vi "FTW-ExtendedActorTemplate.vi"(0 "FTW Actor Instance Configuration":string="{\n  \"Identity\": \"ActorName\",\n  \"InboxAddress\": \"inproc://*\",\n  \"LoggerAddress\": \"\",\n  \"DebugEnableInboxLogging\": false,\n  \"DebugEnableJobLogging\": false,\n  \"LauncherAddress\": \"\",\n  \"Connections\": {\n    \"ConnectionOne\": \"inproc://connection-one\",\n    \"ConnectionTwo\": \"tcp://localhost/connection-two\"\n  },\n  \"Publishers\": {\n    \"PublisherOne\": \"inproc://publisher-one\",\n    \"PublisherTwo\": \"tcp://localhost/publisher-two\"\n  },\n  \"Subscriptions\": {\n    \"SubscriptionOne\": \"inproc://subscription-one\",\n    \"SubscriptionTwo\": \"tcp://localhost/subscription-two\"\n  }\n}", 11 "ErrorIn":errorcluster) -> (15 "Error":errorcluster)   [LabVIEW 2013]
uses:
  source/actor/Instance-Extended/FTW-ActorExtended.lvclass
  source/actor/Message/Base/FTW-Message.lvclass
  source/actor/Instance/FTW-ActorInstance.lvclass/FTW-ActorInstance.ctl
  source/actor/JobSequencer/FTW-SEQ-Current.vi
  source/actor/Instance/FTW-ActorInstance.lvclass
  source/actor/Message/Request/FTW-Message-IncomingRequest.lvclass
panel:
  # "Inputs"
  # "Outputs"
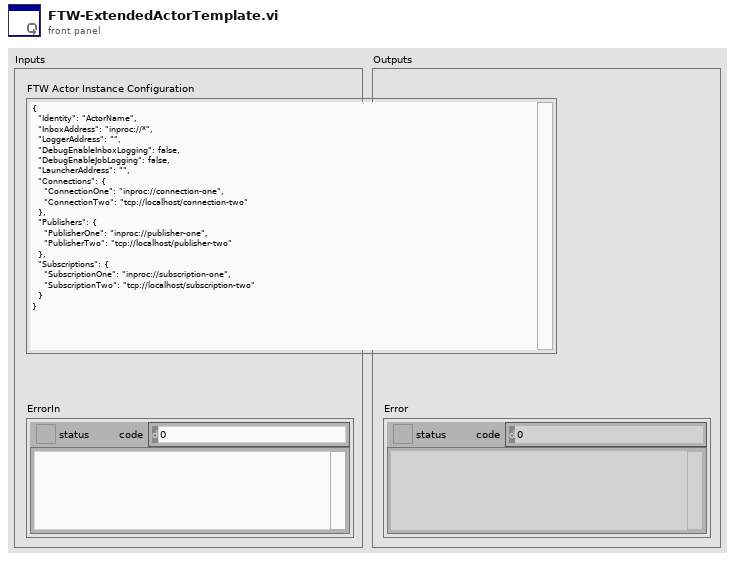
[diagram p1: front panel]
types:
  T1 = cluster{"Incoming Requests":refnum<event-registration>, "Local Messages":refnum<event-registration>, "Subscriber Registration":refnum<event-registration>}
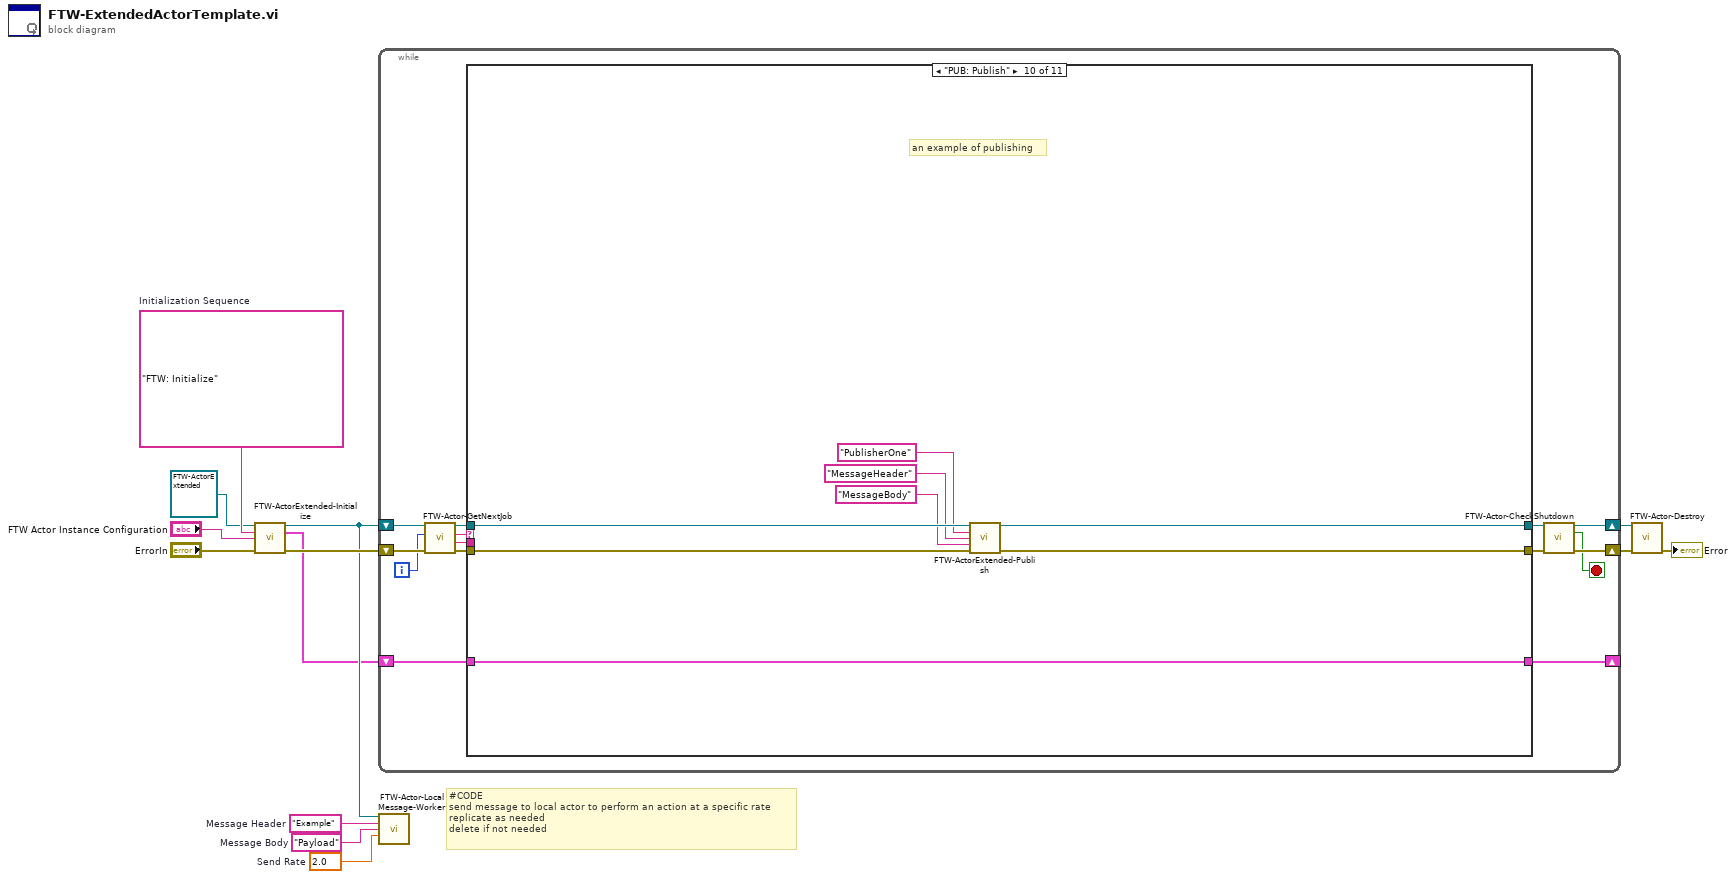
[diagram p0: block diagram]
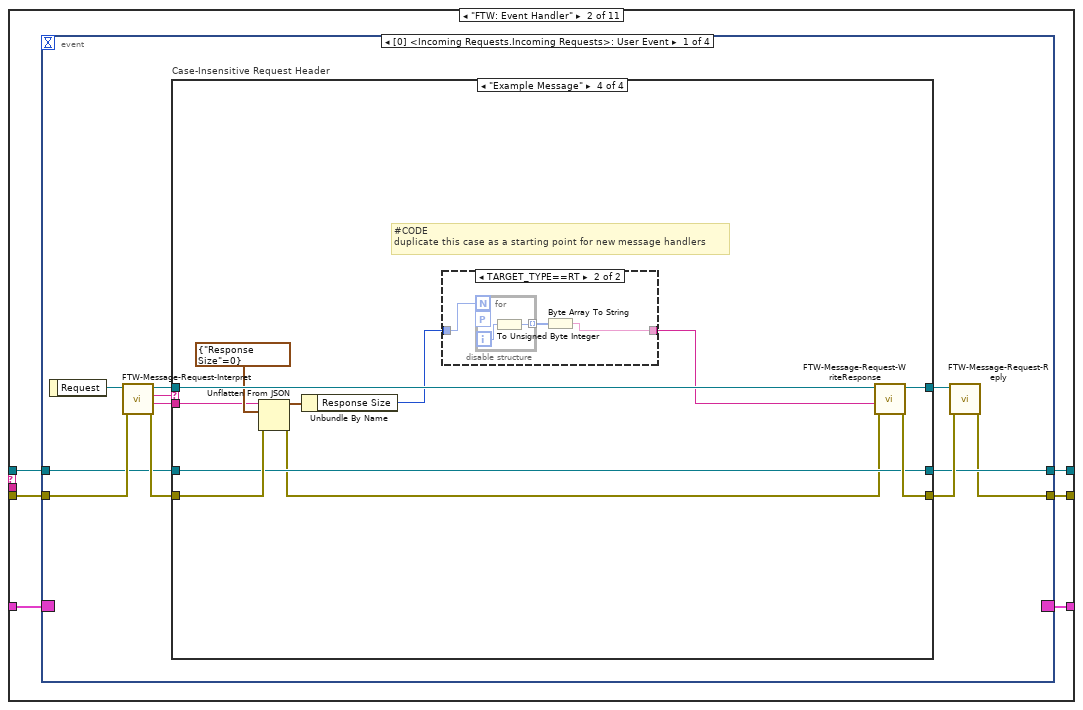
[diagram p3: hidden frame]
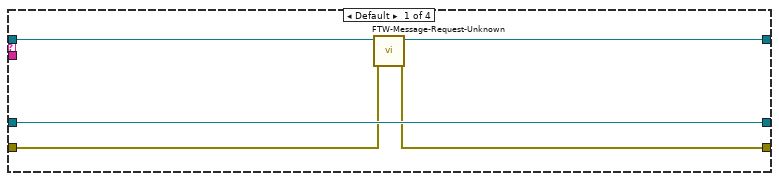
[diagram p4: hidden frame]
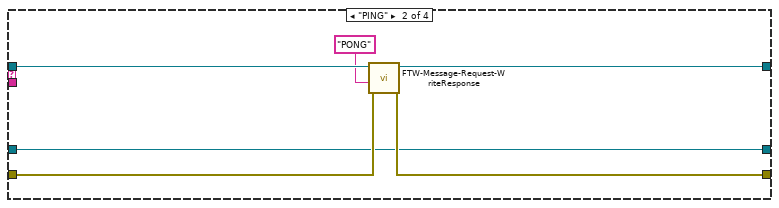
[diagram p5: hidden frame]
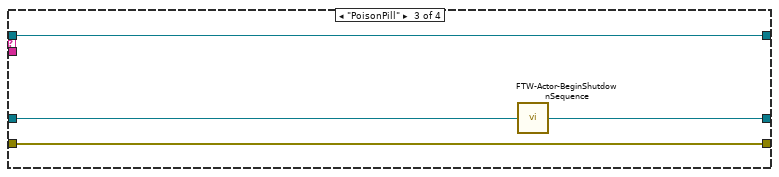
[diagram p6: hidden frame]
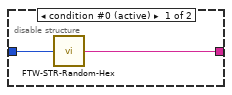
[diagram p7: hidden frame]
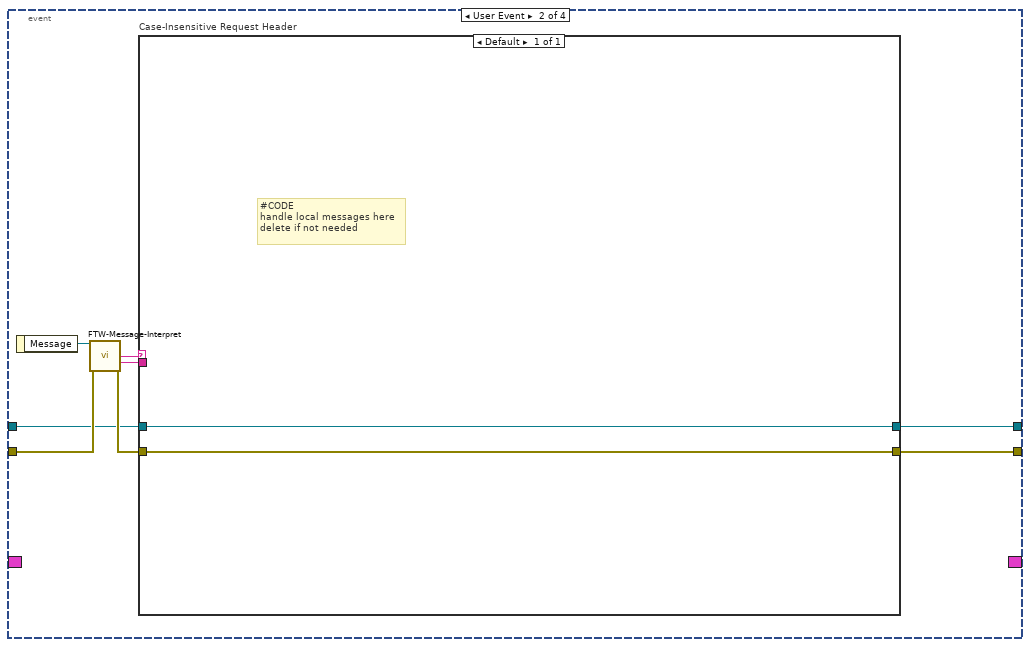
[diagram p8: hidden frame]
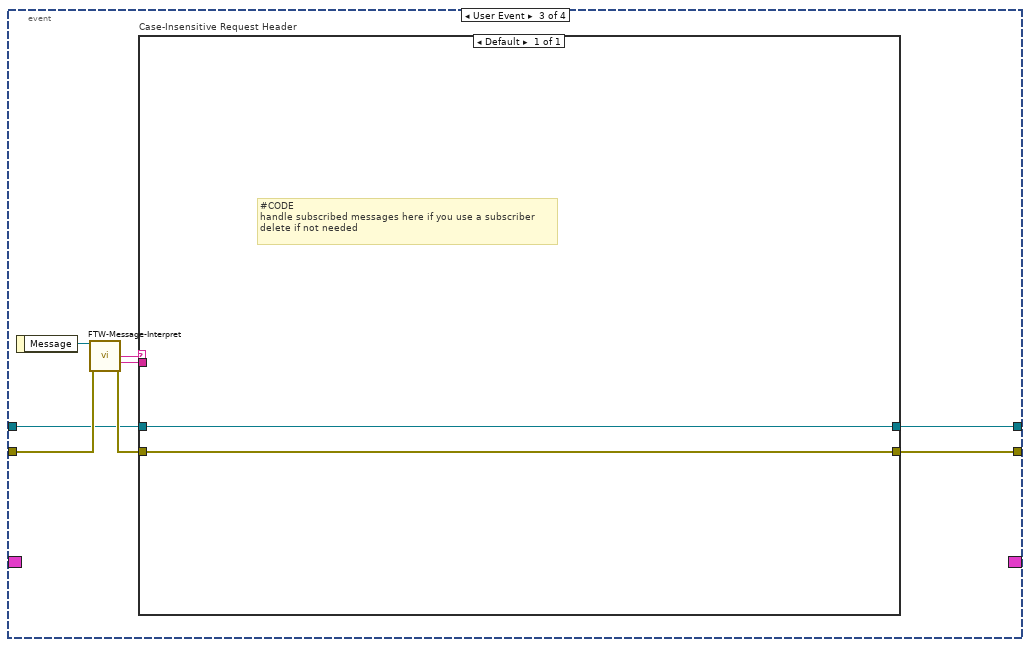
[diagram p9: hidden frame]
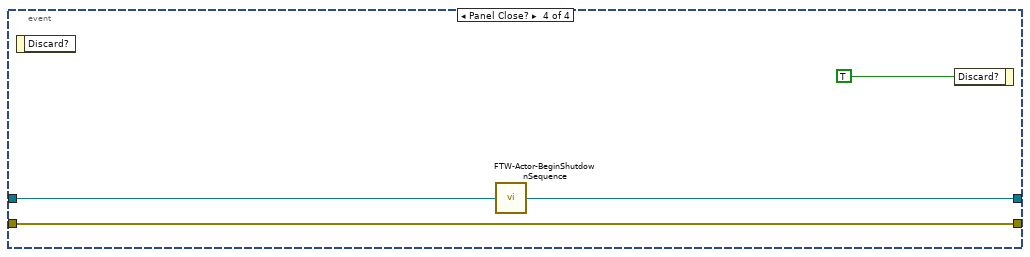
[diagram p10: hidden frame]
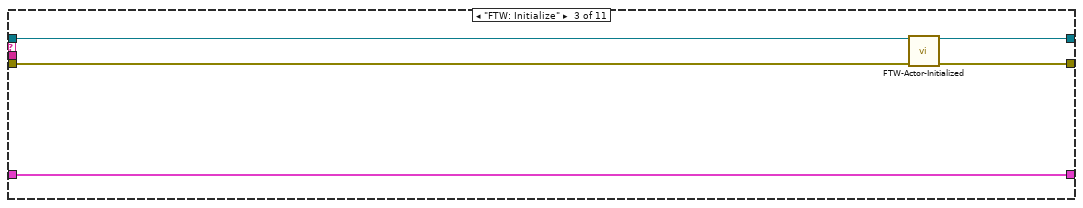
[diagram p11: hidden frame]
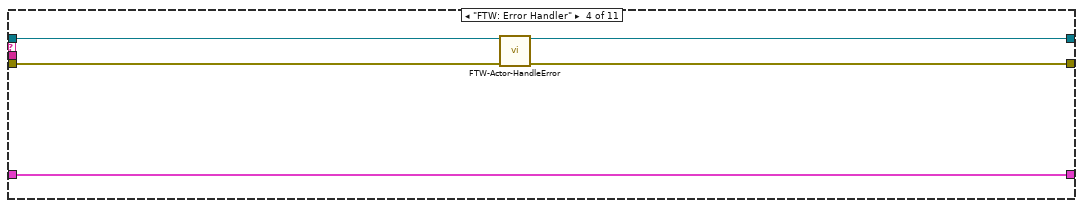
[diagram p12: hidden frame]
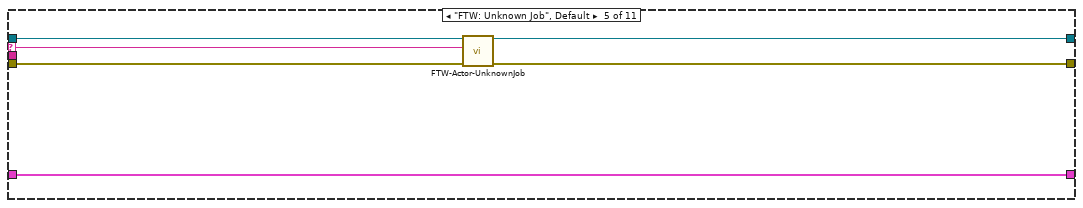
[diagram p13: hidden frame]
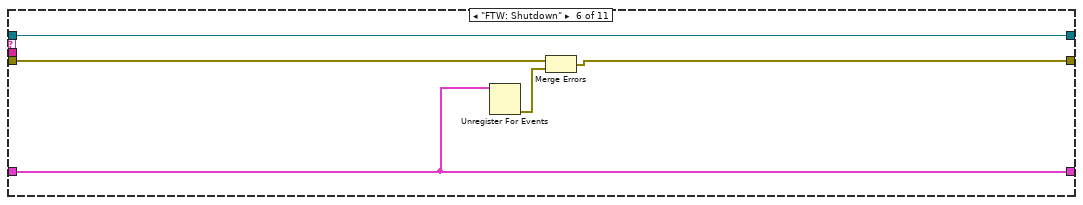
[diagram p14: hidden frame]
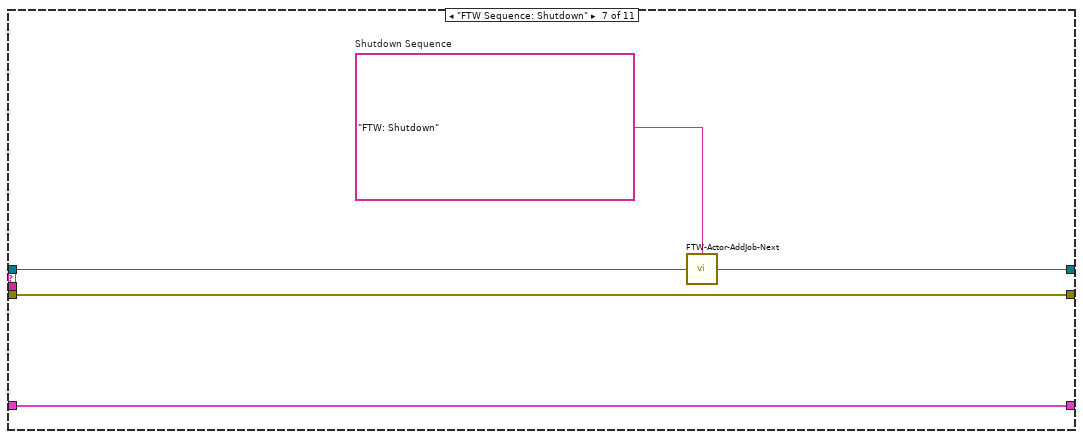
[diagram p15: hidden frame]
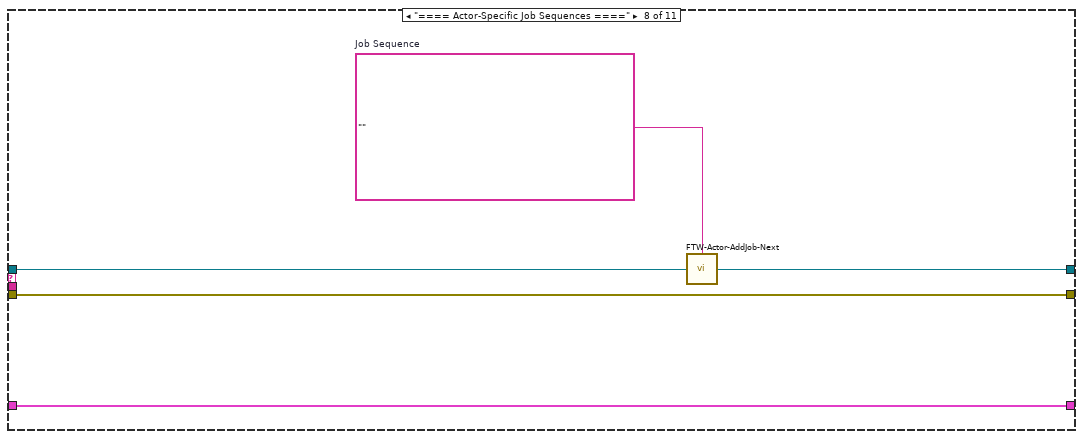
[diagram p16: hidden frame]
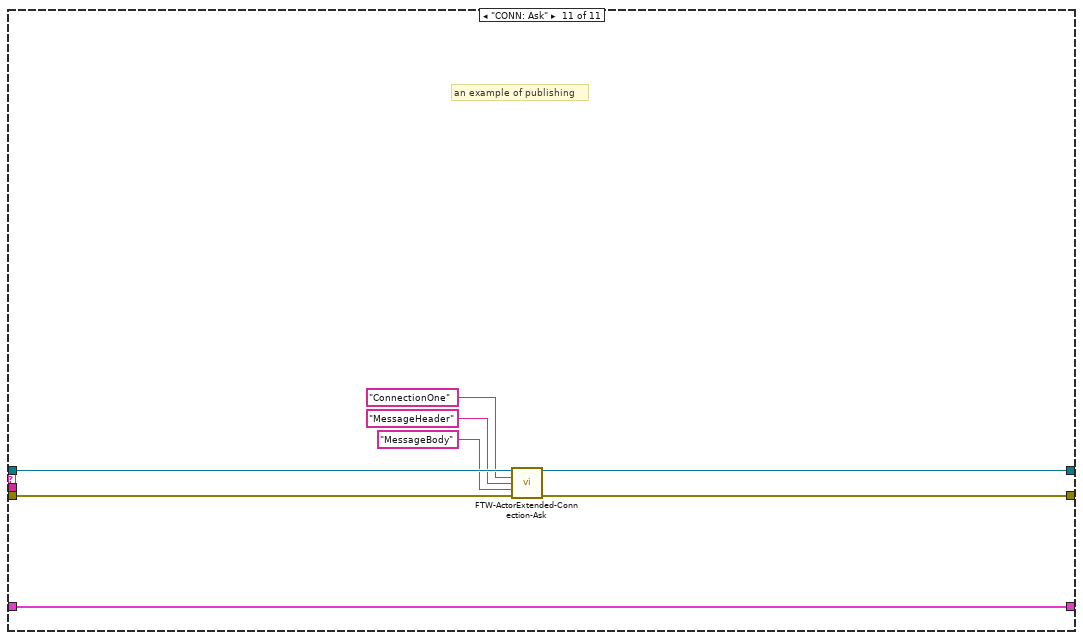
[diagram p18: hidden frame]
diagram:
  w3 = 2.0  # Send Rate
  w4 = "Payload"  # Message Body
  w5 = "Example"  # Message Header
  w9 = "FTW: Initialize"  # Initialization Sequence
  # "#CODE\nsend message to local actor to perform an action at a specific rate\nreplicate as needed\ndelete if not needed"
  n1 = call-dynamic "FTW-ActorExtended-Initialize.vi"("FTW Actor Instance Type"=refnum<class "FTW-ActorExtended.lvclass"> refnum, "Initialization Job Sequence"=w9, "Actor Instance Configuration"="FTW Actor Instance Configuration", "error in"="ErrorIn") -> ("FTW Actor Instance"=w6:refnum<class "FTW-ActorExtended.lvclass">, "Event Refnums"=w2:T1, "error out"=w10:errorcluster)  [unwired: 9 in]
  n2 = while {
    shift-right: [w17] -> w12
    shift-left: w10 -> [w24]
    shift-right: [w14] -> _
    shift-left: w2 -> [w27]
    shift-right: [w19] -> w13
    shift-left: w6 -> [w26]
    i -> [w15]
    stop <- w16 stop-if-true
    n3 = call "FTW-Actor-GetNextJob.vi"("error in"=w24, "Jobs Performed"=w15, "FTW Actor Instance"=w26) -> ("error out"=w23:errorcluster, "Job Data"=w21:string, "Job Name"=w22:string, "FTW Actor Instance out"=w25:refnum<class "FTW-ActorExtended.lvclass">)  [unwired: 5 in]
    n4 = case shown="\"PUB: Publish\"" w22 {
      selector: w22 -> [_ _ _ _ w115 _ _ _ _ _ _]
      tunnel: [w29 w36 w105 w110 w118 w124 w129 w134 w138 w142 w150] -> w18
      tunnel: w23 -> [w29 w35 w108 w112 w119 w125 w129 w134 w138 w143 w151]
      tunnel: w27 -> [w30 w31 w109 w114 w120 w121 w130 w135 w137 w146 w154]
      tunnel: [w30 w34 w109 w114 w120 w121 w130 w135 w137 w146 w154] -> w14
      tunnel: w21 -> [_ _ _ _ _ _ _ _ _ _ _]
      tunnel: [w28 w33 w106 w111 w116 w122 w127 w132 w136 w144 w152] -> w20
      tunnel: w25 -> [w28 w32 w107 w113 w117 w122 w128 w133 w136 w145 w153]
      frame "==== Featherweight Framework Jobs ====" {
      }
      frame "FTW: Event Handler" {
        n5 = event shown="[0] <Incoming Requests.Incoming Requests>: User Event" {
          selector: w31 -> [_ _ _ _]
          dyn-events: [_ _ _ _] -> w34
          timeout: _ -> [_ _ _ _]
          tunnel: [w39 w85 w95 w103] -> w36
          tunnel: w35 -> [w45 w86 w96 w103]
          tunnel: [w43 w84 w94 w101] -> w33
          tunnel: w32 -> [w42 w83 w93 w102]
          event User Event {
            n6 = event-data() -> ("Request"=w46:refnum<class "FTW-Message-IncomingRequest.lvclass">)  [unwired: 1 in]
            n7 = call "FTW-Message-Request-Interpret.vi"("error in"=w45, "FTW Incoming Request"=w46) -> ("error out"=w47:errorcluster, "Request Body"=w37:string, "Request Header"=w41:string, "FTW Incoming Request out"=w40:refnum<class "FTW-Message-IncomingRequest.lvclass">)  [unwired: 6 in]
            n8 = case "Case-Insensitive Request Header" shown="\"Example Message\"" w41 {
              tunnel: [w50 w56 w61 w72] -> w44
              tunnel: w47 -> [w51 w57 w61 w73]
              tunnel: [w52 w55 w62 w69] -> w43
              tunnel: w42 -> [w52 w55 w60 w69]
              tunnel: w40 -> [w49 w58 w59 w71]
              tunnel: [w48 w54 w59 w70] -> w38
              tunnel: w37 -> [_ _ _ w63]
              frame Default {
                n9 = call "FTW-Message-Request-Unknown.vi"("error in"=w51, "FTW Incoming Request"=w49) -> ("error out"=w50:errorcluster, "FTW Incoming Request Out"=w48:refnum<class "FTW-Message-IncomingRequest.lvclass">)  [unwired: 8 in]
              }
              frame "PING" {
                n10 = call "FTW-Message-Request-WriteResponse.vi"("error in"=w57, "Response Body"="PONG" ("Response Header"), "FTW Incoming Request"=w58) -> ("error out"=w56:errorcluster, "FTW Incoming Request out"=w54:refnum<class "FTW-Message-IncomingRequest.lvclass">)  [unwired: 7 in]
              }
              frame "PoisonPill" {
                n11 = call "FTW-Actor-BeginShutdownSequence.vi"("FTW Actor Instance"=w60) -> ("FTW Actor Instance out"=w62:refnum<class "FTW-ActorExtended.lvclass">)  [unwired: 3 in]
              }
              frame "Example Message" {
                # "#CODE\nduplicate this case as a starting point for new message handlers"
                n12 = Unflatten From JSON(JSON string=w63, type and defaults=cluster{"Response Size":i32} {"Response Size"=0}, error in (no error)=w73) -> (value=w66:cluster{"Response Size":i32}, error out=w68:errorcluster)  [unwired: 4 in]
                n13 = Unbundle By Name(w66) -> ("Response Size"=w65:i32)
                n14 = disable-structure shown="TARGET_TYPE==RT" {
                  disable-tunnel: w65 -> [w75 w78]
                  disable-tunnel: [w74 w76] -> w64
                  frame condition #0 (active) {
                    n15 = call "FTW-STR-Random-Hex.vi"("String Length"=w75) -> ("Random Hex String"=w74:string)  [unwired: 3 in]
                  }
                  frame condition #1 {
                    n16 = for {
                      N: w78 -> [_]
                      workers-P: _ -> [_]
                      tunnel: [w79] -> w77 mode=indexing
                      i -> [w80]
                      n17 = To Unsigned Byte Integer(number=w80) -> (unsigned 8bit integer=w79:u8)
                    }
                    n18 = Byte Array To String(unsigned byte array=w77) -> (string=w76:string)
                  }
                }
                n19 = call "FTW-Message-Request-WriteResponse.vi"("error in"=w68, "Response Body"=w64, "FTW Incoming Request"=w71) -> ("error out"=w72:errorcluster, "FTW Incoming Request out"=w70:refnum<class "FTW-Message-IncomingRequest.lvclass">)  [unwired: 7 in]
              }
            }
            n20 = call "FTW-Message-Request-Reply.vi"("FTW: Reply Error"=w44, "FTW Incoming Request"=w38) -> ("error out"=w39:errorcluster)  [unwired: 8 in, 1 out]
          }
          event User Event {
            n21 = event-data() -> ("Message"=w87:refnum<class "FTW-Message.lvclass">)  [unwired: 1 in]
            n22 = call-dynamic "FTW-Message-Interpret.vi"("FTW Message"=w87, "error in"=w86) -> ("Message Header"=w81:string, "Message Body"=w82:string, "error out"=w88:errorcluster)  [unwired: 9 in, 2 out]
            n23 = case "Case-Insensitive Request Header" shown="Default" w81 {
              tunnel: [w89] -> w85
              tunnel: w88 -> [w89]
              tunnel: [w90] -> w84
              tunnel: w83 -> [w90]
              tunnel: w82 -> [_]
              frame Default {
                # "#CODE\nhandle local messages here\ndelete if not needed"
              }
            }
          }
          event User Event {
            n24 = event-data() -> ("Message"=w97:refnum<class "FTW-Message.lvclass">)  [unwired: 1 in]
            n25 = call-dynamic "FTW-Message-Interpret.vi"("FTW Message"=w97, "error in"=w96) -> ("Message Header"=w91:string, "Message Body"=w92:string, "error out"=w98:errorcluster)  [unwired: 9 in, 2 out]
            n26 = case "Case-Insensitive Request Header" shown="Default" w91 {
              tunnel: [w99] -> w95
              tunnel: w98 -> [w99]
              tunnel: [w100] -> w94
              tunnel: w93 -> [w100]
              tunnel: w92 -> [_]
              frame Default {
                # "#CODE\nhandle subscribed messages here if you use a subscriber\ndelete if not needed"
              }
            }
          }
          event Panel Close? {
            n27 = event-data() -> ()  [unwired: 1 in, 1 out]
            n28 = call "FTW-Actor-BeginShutdownSequence.vi"("FTW Actor Instance"=w102) -> ("FTW Actor Instance out"=w101:refnum<class "FTW-ActorExtended.lvclass">)  [unwired: 3 in]
            n29 = event-data("Discard?"=TRUE) -> ()  [unwired: 1 in, 1 out]
          }
        }
      }
      frame "FTW: Initialize" {
        n30 = call-dynamic "FTW-Actor-Initialized.vi"("FTW Actor Instance"=w107, "error in"=w108) -> ("FTW Actor Instance out"=w106:refnum<class "FTW-ActorExtended.lvclass">, "error out"=w105:errorcluster)  [unwired: 12 in]
      }
      frame "FTW: Error Handler" {
        n31 = call-dynamic "FTW-Actor-HandleError.vi"("FTW Actor Instance"=w113, "error in"=w112) -> ("FTW Actor Instance out"=w111:refnum<class "FTW-ActorExtended.lvclass">, "error out"=w110:errorcluster)  [unwired: 10 in, 2 out]
      }
      frame "FTW: Unknown Job", Default {
        n32 = call-dynamic "FTW-Actor-UnknownJob.vi"("FTW Actor Instance"=w117, "Unknown Job"=w115, "error in"=w119) -> ("FTW Actor Instance out"=w116:refnum<class "FTW-ActorExtended.lvclass">, "error out"=w118:errorcluster)  [unwired: 11 in]
      }
      frame "FTW: Shutdown" {
        n33 = Unregister For Events(event registration refnum=w121) -> (error out=w123:errorcluster)  [unwired: 1 in]
        n34 = Merge Errors(w125, w123) -> (w124:errorcluster)
      }
      frame "FTW Sequence: Shutdown" {
        w126 = "FTW: Shutdown"  # Shutdown Sequence
        n35 = call "FTW-Actor-AddJob-Next.vi"("Add Next in Job Queue"=w126, "FTW Actor Instance"=w128) -> ("FTW Actor Instance out"=w127:refnum<class "FTW-ActorExtended.lvclass">)  [unwired: 2 in]
      }
      frame "==== Actor-Specific Job Sequences ====" {
        w131 = ""  # Job Sequence
        n36 = call "FTW-Actor-AddJob-Next.vi"("Add Next in Job Queue"=w131, "FTW Actor Instance"=w133) -> ("FTW Actor Instance out"=w132:refnum<class "FTW-ActorExtended.lvclass">)  [unwired: 2 in]
      }
      frame "==== Actor-Specific Jobs ====" {
      }
      frame "PUB: Publish" {
        # "an example of publishing"
        n37 = call "FTW-ActorExtended-Publish.vi"("FTW-ActorExtended In"=w145, "Publisher Name"="PublisherOne", "Message Header"="MessageHeader", "Message Body"="MessageBody", "error in"=w143) -> ("FTW-ActorExtended Out"=w144:refnum<class "FTW-ActorExtended.lvclass">, "error out"=w142:errorcluster)  [unwired: 9 in]
      }
      frame "CONN: Ask" {
        # "an example of publishing"
        n38 = call "FTW-ActorExtended-Connection-Ask.vi"("FTW-ActorExtended In"=w153, "Connector Name"="ConnectionOne" ("Publisher Name"), "Message Header"="MessageHeader", "Message Body"="MessageBody", "error in"=w151) -> ("FTW-ActorExtended Out"=w152:refnum<class "FTW-ActorExtended.lvclass">, "error out"=w150:errorcluster)  [unwired: 5 in, 4 out]
      }
    }
    n39 = call "FTW-Actor-CheckShutdown.vi"("FTW Actor Instance"=w20, "error in"=w18) -> ("FTW Actor Instance out"=w19:refnum<class "FTW-ActorExtended.lvclass">, "Shutdown?"=w16:bool, "error out"=w17:errorcluster)  [unwired: 11 in]
  }
  n40 = call-dynamic "FTW-Actor-LocalMessage-Worker.vi"("FTW-ActorInstance In"=w6, "Message Header"=w5, "Message Body"=w4, "Send Rate"=w3) -> ()  [unwired: 12 in]
  n41 = call-dynamic "FTW-Actor-Destroy.vi"("FTW Actor Instance"=w13, "error in"=w12) -> ("error out"=→"Error":errorcluster)  [unwired: 13 in]
